vi "Run Tx - Handle Transmit Option.vi"(8 "error in (no error)":errorcluster, 10 "Transmit Flag":T2, 11 "Transmit Option":T1) -> (0 "error out":errorcluster, 3 "Transmit?":bool, 5 "Transmit Values":dbl[](array[numeric]))   [LabVIEW 2021, in "UDP-Custom-Device Engine.lvlib"]
uses:
  UDP-Custom-Device Engine.lvlib
  <vilib>/NI/NIVS Inline Async API/_Data Access Engine/Data Access Engine/Types/Read.DVR.ctl
  <vilib>/NI/NIVS Inline Async API/_Data Access Engine/Access Type Classes/Read/Read.lvclass
  Shared/Types/Shared - Transmit Flag Options.ctl
  <vilib>/NI/NIVS Inline Async API/_Data Access Engine/Access Type Classes/Read/Read.lvclass/Read.ctl
  <vilib>/NI/NIVS Inline Async API/_Data Access Engine/Data Access Engine/Methods/Read.Data.vi
  <vilib>/NI/NIVS Inline Async API/_Data Access Engine/Access Type Classes/Read/Read.ProcessData.vi
  <vilib>/NI/NIVS Inline Async API/_Data Access Engine/Data Access Engine/Data Access Engine.lvclass
  Shared/UDP-Custom-Device Shared.lvlib
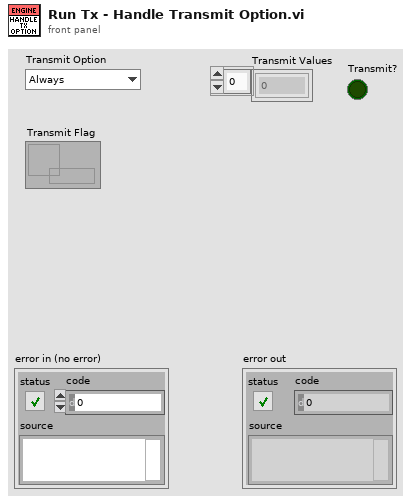
[diagram p1: front panel]
types:
  T1 = typedef "UDP-Custom-Device Shared.lvlib/Shared - Transmit Flag Options.ctl" = enum16{"Always", "One-Shot", "Toggle"}
  T2 = typedef "Data Access Engine.lvlib/Data Access Engine.lvclass/Read.DVR.ctl" = refnum<data-value>
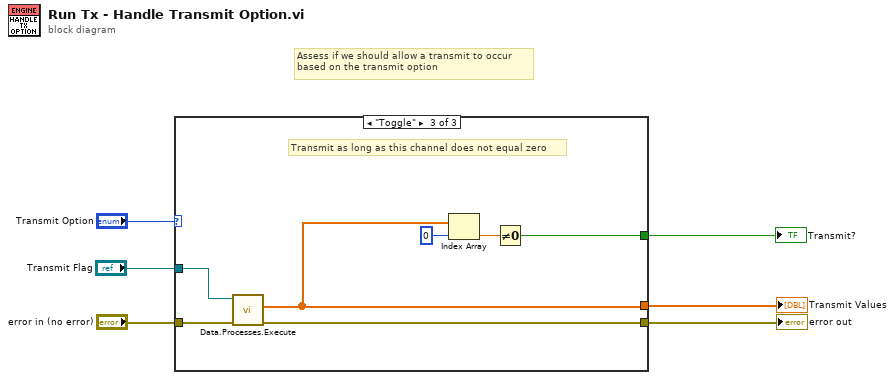
[diagram p0: block diagram]
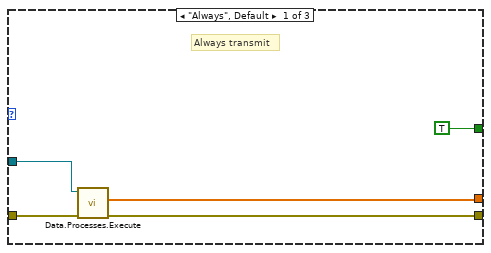
[diagram p2: hidden frame]
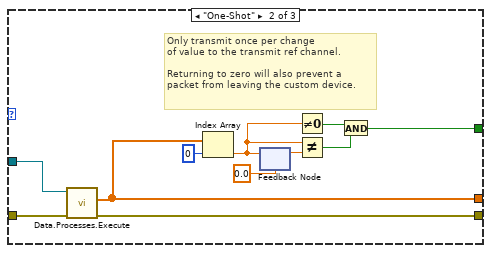
[diagram p3: hidden frame]
diagram:
  # "Assess if we should allow a transmit to occur\nbased on the transmit option"
  n1 = case shown="\"Toggle\"" "Transmit Option" {
    tunnel: [w9 w13 w24] -> w2
    tunnel: "error in (no error)" -> [w10 w21 w28]
    tunnel: [TRUE w15 w25] -> w4
    tunnel: "Transmit Flag" -> [w8 w20 w27]
    tunnel: [w7 w12 w23] -> w1
    frame "Always", Default {
      # "Always transmit"
      n2 = call-poly <vilib>:"Data.Processes.Execute.vi"("error in (no error)"=w10, "Ref"=w8) -> ("error out"=w9:errorcluster, "Values"=w7:dbl[])  [unwired: 7 in, 1 out]
    }
    frame "One-Shot" {
      # "Only transmit once per change\nof value to the transmit ref channel.\n\nReturning to zero will also prevent a\npacket from leaving the custom device."
      n3 = call-poly <vilib>:"Data.Processes.Execute.vi"("error in (no error)"=w21, "Ref"=w20) -> ("error out"=w13:errorcluster, "Values"=w12:dbl[])  [unwired: 7 in, 1 out]
      n4 = Index Array(array=w12, index=0) -> (element=w18:dbl)
      n5 = feedback-in #1(w18) -> ()
      n6 = feedback #1(0.0 ("Channel Data Reference")) -> (w19:dbl)
      n7 = Not Equal To 0?(x=w18) -> (x != 0?=w17:bool)
      n8 = Not Equal?(x=w18, y=w19) -> (x != y?=w16:bool)
      n9 = And(x=w17, y=w16) -> (x .and. y?=w15:bool)
    }
    frame "Toggle" {
      # "Transmit as long as this channel does not equal zero"
      n10 = call-poly <vilib>:"Data.Processes.Execute.vi"("error in (no error)"=w28, "Ref"=w27) -> ("error out"=w24:errorcluster, "Values"=w23:dbl[])  [unwired: 7 in, 1 out]
      n11 = Index Array(array=w23, index=0) -> (element=w26:dbl)
      n12 = Not Equal To 0?(x=w26) -> (x != 0?=w25:bool)
    }
  }
  "error out" <- w2
  "Transmit?" <- w4
  "Transmit Values" <- w1
